vi "execution class name.vi"(8 "error in":errorcluster, 11 "configuration in":refnum<class "TBM module configuration.lvclass">) -> (0 "error out":errorcluster, 2 "execution class":string, 3 "configuration out":refnum<class "TBM module configuration.lvclass">)   [LabVIEW 2013, in "TBM module configuration.lvclass"]
uses:
  TBM module configuration.lvclass
  root configuration/TBM configuration.lvclass
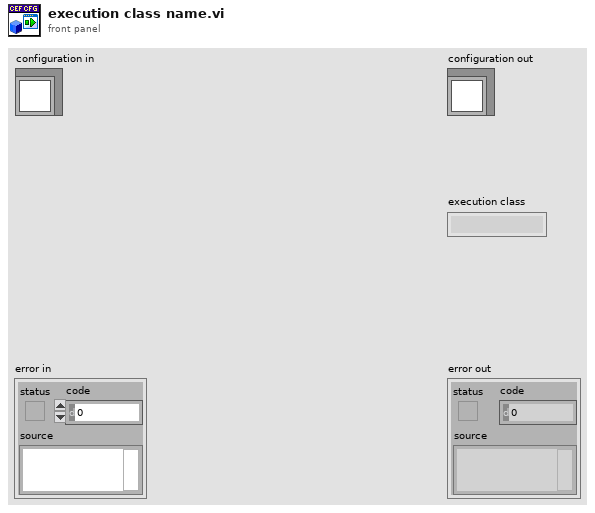
[diagram p1: front panel]
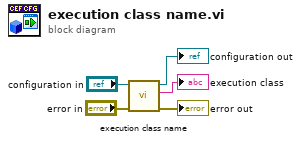
[diagram p0: block diagram]
diagram:
  n1 = call-parent "execution class name.vi"("error in"="error in", "configuration in"="configuration in") -> ("error out"=→"error out":errorcluster, "execution class"=→"execution class":string, "configuration out"=→"configuration out":refnum<class "TBM module configuration.lvclass">)  [unwired: 7 in]
